vi "get_power_level.vi"(8 "error in (no error)":errorcluster, 10 "Layer":u8, 11 "VISA resource name":refnum<visa-resource-name>) -> (0 "error out":errorcluster, 2 "Power (%)":sgl format="%#_13g", 3 "VISA resource name out":refnum<visa-resource-name>)   [LabVIEW 2018]
doc: "Start the active process or continue a process that is in the STOP state."
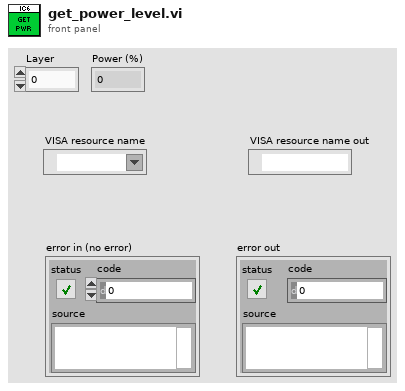
[diagram p1: front panel]
types:
  T1 = enum16{"Source", "General", "Input name", "Process name", "Logic", "Material", "Material name", "Output name", "Process", "Sensor", "Output type", "User message", "Layer", ""}
  T2 = enum16{"Hello", "Query", "Remote action", "Status", "Update"}
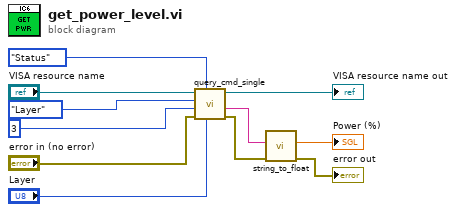
[diagram p0: block diagram]
diagram:
  n1 = call "query_cmd_single.vi"("Parameter"="Layer", "Command group"=T2."Status", "error in (no error)"="error in (no error)", "Command ID"=u8 3, "Command subgroup"=T1."Layer", "VISA resource name"="VISA resource name") -> ("error out"=w3:errorcluster, "formatted response"=w4:string, "VISA resource name out"=→"VISA resource name out":refnum<visa-resource-name>)  [unwired: 1 in, 2 out]
  n2 = call "string_to_float.vi"("error in (no error)"=w3, "Float (string)"=w4) -> ("error out"=→"error out":errorcluster, "Float (sgl)"=→"Power (%)":sgl)  [unwired: 8 in]
